vi "Copy From Diagram to Private Data.vi"(6 "Add as Reference?":bool, 8 "error in (no error)":errorcluster, 9 "Text to Append (\" Ref\")":string=" Ref", 10 "GObjects in":refnum<vi>[](array[refnum]), 11 "Private Data Refs":T1) -> (0 "error out":errorcluster, 2 "Other GObjects":refnum<vi>[](array[refnum]), 3 "ControlReferenceConstants":refnum<vi>[](array[refnum]))   [LabVIEW 2020, in "Add to Private Data.lvlib"]
uses:
  Add to Private Data.lvlib
  Private Data Refs.ctl
  <vilib>/regexp/Match Regular Expression.xnode
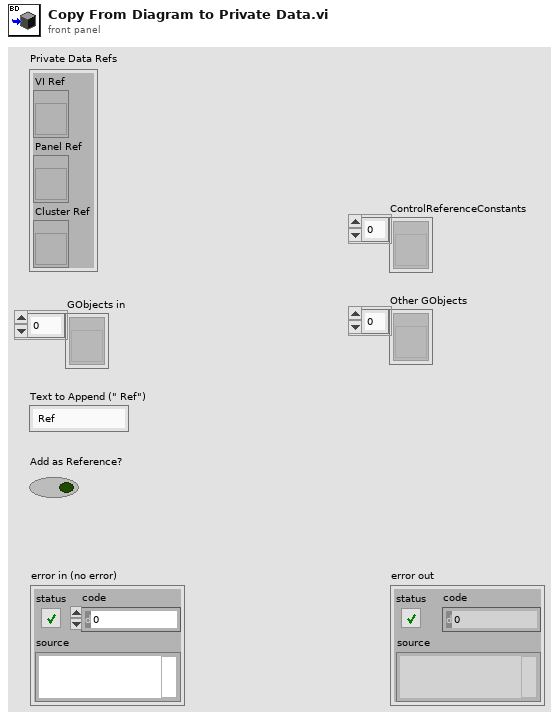
[diagram p1: front panel]
types:
  T1 = typedef "Add to Private Data.lvlib/Private Data Refs.ctl" = cluster{"VI Ref":refnum<vi>, "Panel Ref":refnum<vi>, "Cluster Ref":refnum<vi>}
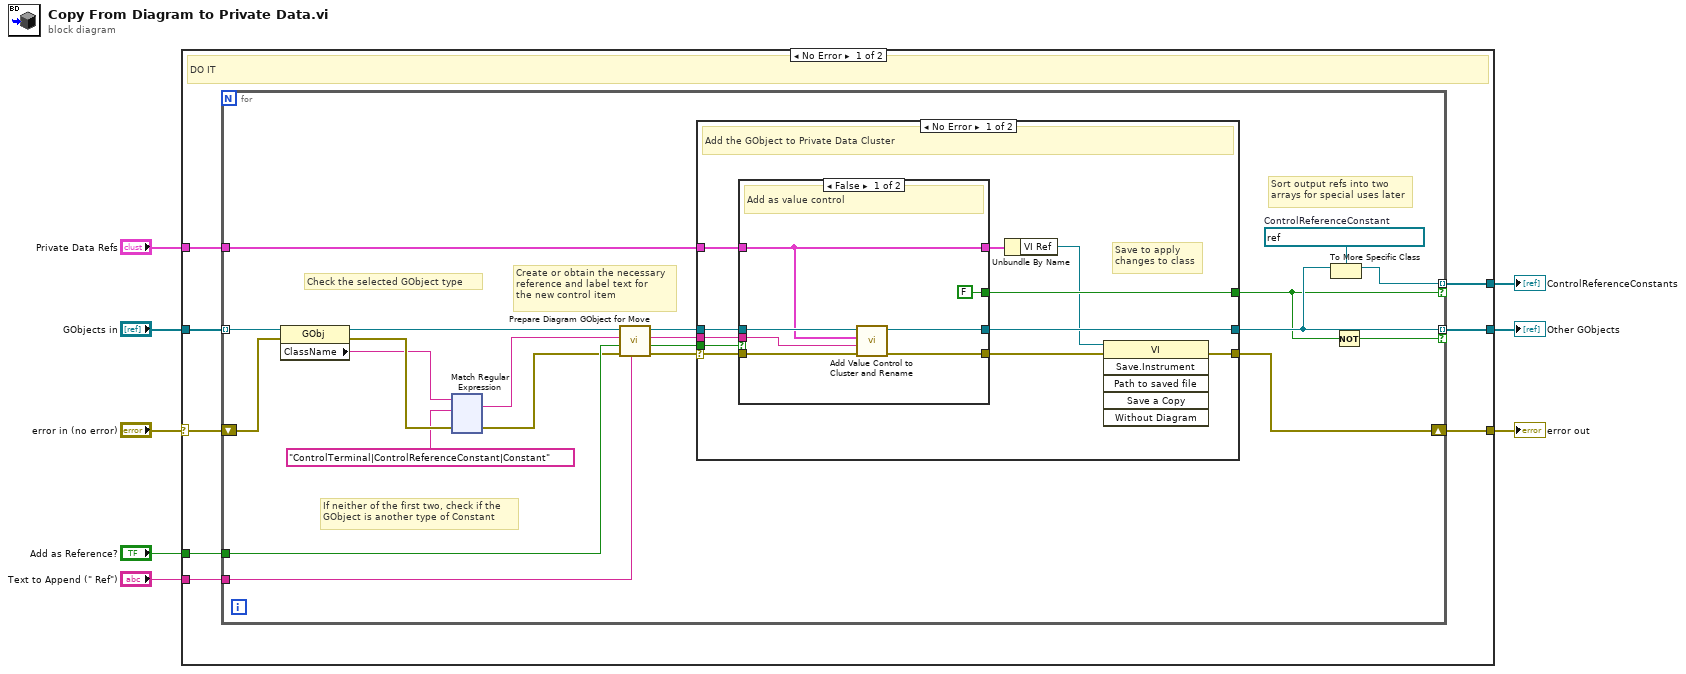
[diagram p0: block diagram]
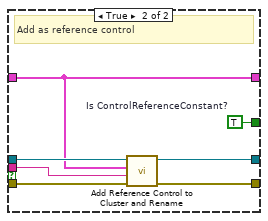
[diagram p2: hidden frame]
diagram:
  n1 = case shown="No Error" "error in (no error)" {
    selector: "error in (no error)" -> [w9 w179]
    tunnel: [w16 w179] -> w8
    tunnel: "GObjects in" -> [w15 w178]
    tunnel: "Text to Append (\" Ref\")" -> [w14 _]
    tunnel: "Private Data Refs" -> [w13 _]
    tunnel: "Add as Reference?" -> [w12 _]
    tunnel: [w11 w178] -> w3
    tunnel: [w10 _] -> w2
    frame No Error {
      # "DO IT"
      n2 = for {
        tunnel: w15 -> [w35] mode=indexing
        tunnel: w14 -> [w33]
        tunnel: w13 -> [w17]
        shift-right: [w18] -> w16
        shift-left: w9 -> [w34]
        tunnel: w12 -> [w32]
        tunnel: [w23] -> w11 mode=indexing if=w22
        tunnel: [w20] -> w10 mode=indexing if=w21
        w19 = refnum<vi> refnum  # ControlReferenceConstant
        # "Sort output refs into two\narrays for special uses later"
        # "Check the selected GObject type"
        # "If neither of the first two, check if the\nGObject is another type of Constant"
        # "Create or obtain the necessary\nreference and label text for\nthe new control item"
        n3 = property on="Property Node" class="GObj"(reference=w35, error in=w34) -> (reference out=w36:refnum<vi>, error out=w37:errorcluster, "ClassName"=w31:string)
        n4 = xnode "Match Regular Expression"("input string"=w31, "regular expression"="ControlTerminal|ControlReferenceConstant|Constant", "error in"=w37) -> ("whole match"=w30:string, "error out"=w26:errorcluster)  [unwired: 3 in, 3 out]
        n5 = call "Prepare Diagram GObject for Move.vi"("Reference Text to Append (\" Ref\")"=w33, "error in (no error)"=w26, "Add as Reference?"=w32, "Parsed GObject Class Name"=w30, "GObject in"=w36) -> ("error out"=w25:errorcluster, "Updated Add as Reference?"=w24:bool, "Label.Text"=w28:string, "GObject out"=w29:refnum<vi>)  [unwired: 3 in]
        n6 = case shown="No Error" w25 {
          selector: w25 -> [w44 _]
          tunnel: [w40 _] -> w18
          tunnel: w17 -> [w47 _]
          tunnel: w29 -> [w46 w63]
          tunnel: w28 -> [w45 _]
          tunnel: w24 -> [w43 _]
          tunnel: [w42 w63] -> w23
          tunnel: [w41 _] -> w21
          frame No Error {
            # "Save to apply\nchanges to class"
            # "Add the GObject to Private Data Cluster"
            n7 = case shown="False" w43 {
              tunnel: [w55 w61] -> w48
              tunnel: w46 -> [w52 w60]
              tunnel: w44 -> [w54 w62]
              tunnel: w47 -> [w49 w56]
              tunnel: w45 -> [w53 w59]
              tunnel: [w51 w58] -> w42
              tunnel: [FALSE w57] -> w41
              tunnel: [w49 w56] -> w39
              frame False {
                # "Add as value control"
                n8 = call "Add Value Control to Cluster and Rename.vi"("error in (no error)"=w54, "New Label.Text"=w53, "Private Data Refs"=w49, "GObject in"=w52) -> ("error out"=w55:errorcluster, "GObject out"=w51:refnum<vi>)  [unwired: 6 in]
              }
              frame True {
                w57 = TRUE  # Is ControlReferenceConstant?
                # "Add as reference control"
                n9 = call "Add Reference Control to Cluster and Rename.vi"("error in (no error)"=w62, "New Label.Text"=w59, "Private Data Refs"=w56, "GObject in"=w60) -> ("error out"=w61:errorcluster, "GObject out"=w58:refnum<vi>)  [unwired: 6 in]
              }
            }
            n10 = Unbundle By Name(w39) -> ("VI Ref"=w38:refnum<vi>)
            n11 = invoke class="VI" method="Save.Instrument"(reference=w38, error in=w48) -> (error out=w40:errorcluster)  [unwired: 4 in, 5 out]
          }
          frame Error {
            # "Unhandled type -- ignore it and clear error"
          }
        }
        n12 = To More Specific Class(target class=w19, reference=w23) -> (specific class reference=w20:refnum<vi>)  [unwired: 1 in, 1 out]
        n13 = Not(x=w21) -> (.not. x?=w22:bool)
      }
    }
    frame Error {
      # "Calling VI is probably not a class member."
    }
  }
  "error out" <- w8
  "Other GObjects" <- w3
  "ControlReferenceConstants" <- w2
